vi "Write Data.vi"(8 "error in (no error)":errorcluster, 10 "Data":u16, 11 "Write to Module Msg in":refnum<class "Write to Module Msg.lvclass">) -> (0 "error out":errorcluster, 3 "Write to Module Msg out":refnum<class "Write to Module Msg.lvclass">)   [LabVIEW 2020, in "Modbus.lvlib" / "Write to Module Msg.lvclass"]
uses:
  Write to Module Msg.lvclass
  Write to Module Msg.lvclass/Write to Module Msg.ctl
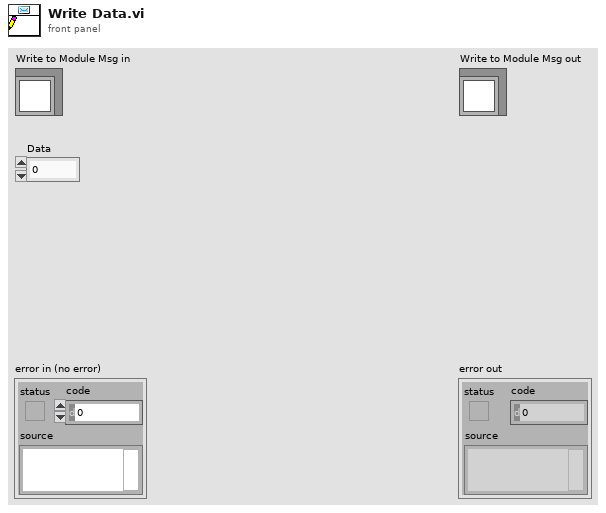
[diagram p1: front panel]
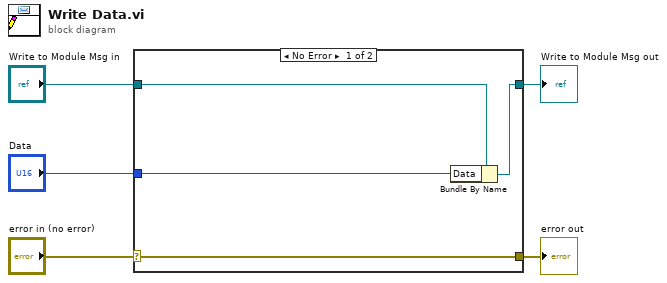
[diagram p0: block diagram]
diagram:
  n1 = case shown="No Error" "error in (no error)" {
    selector: "error in (no error)" -> [w9 w10]
    tunnel: [w9 w10] -> w4
    tunnel: [w7 w11] -> w2
    tunnel: "Write to Module Msg in" -> [w8 w11]
    tunnel: "Data" -> [w6 _]
    frame No Error {
      n2 = Bundle By Name(cluster=w8, "Data"=w6) -> (w7:refnum<class "Write to Module Msg.lvclass">)
    }
    frame Error {
    }
  }
  "error out" <- w4
  "Write to Module Msg out" <- w2
